vi "Convert Metadata Response to V1.vi"(8 "error in":errorcluster, 10 "get metadata response generic in":T10) -> (0 "error out":errorcluster, 2 "get metadata response v1 out":T1)   [LabVIEW 2020, in "Measurement Plugin Measurement Server.lvlib" / "Measurement Service V1.lvclass"]
uses:
  Measurement Service V1.lvclass
  Helpers/TypeDefs/Get Metadata Response.ctl
  Helpers/TypeDefs/Measurement Details.ctl
  Helpers/TypeDefs/Measurement Signature.ctl
  Helpers/TypeDefs/Configuration Parameter.ctl
  Helpers/TypeDefs/Parameter Annotations Entry.ctl
  <vilib>/gRPC/LabVIEW gRPC Library/Shared/Any.ctl
  Helpers/TypeDefs/Output Parameter.ctl
  Helpers/TypeDefs/User Interface Details.ctl
  Generated/Measurement Plugin Measurement Server Internal/RPC Messages/ni_measurementlink_measurement_v1_GetMetadataResponse.ctl
  Generated/Measurement Plugin Measurement Server Internal/RPC Messages/ni_measurementlink_measurement_v1_MeasurementDetails.ctl
  Generated/Measurement Plugin Measurement Server Internal/RPC Messages/ni_measurementlink_measurement_v1_MeasurementSignature.ctl
  Generated/Measurement Plugin Measurement Server Internal/RPC Messages/ni_measurementlink_measurement_v1_ConfigurationParameter.ctl
  Generated/Measurement Plugin Measurement Server Internal/RPC Messages/google_protobuf_Field_Kind.ctl
  Generated/Measurement Plugin Measurement Server Internal/RPC Messages/ni_measurementlink_measurement_v1_ConfigurationParameter_AnnotationsEntry.ctl
  Generated/Measurement Plugin Measurement Server Internal/RPC Messages/google_protobuf_Any.ctl
  Generated/Measurement Plugin Measurement Server Internal/RPC Messages/ni_measurementlink_measurement_v1_Output.ctl
  Generated/Measurement Plugin Measurement Server Internal/RPC Messages/ni_measurementlink_measurement_v1_UserInterfaceDetails.ctl
  Generated/Measurement Plugin Measurement Server Internal/Measurement Plugin Measurement Server Internal.lvlib
  Measurement Plugin Measurement Server.lvlib
  <vilib>/gRPC/LabVIEW gRPC Library/grpc-lvsupport-release.lvlib
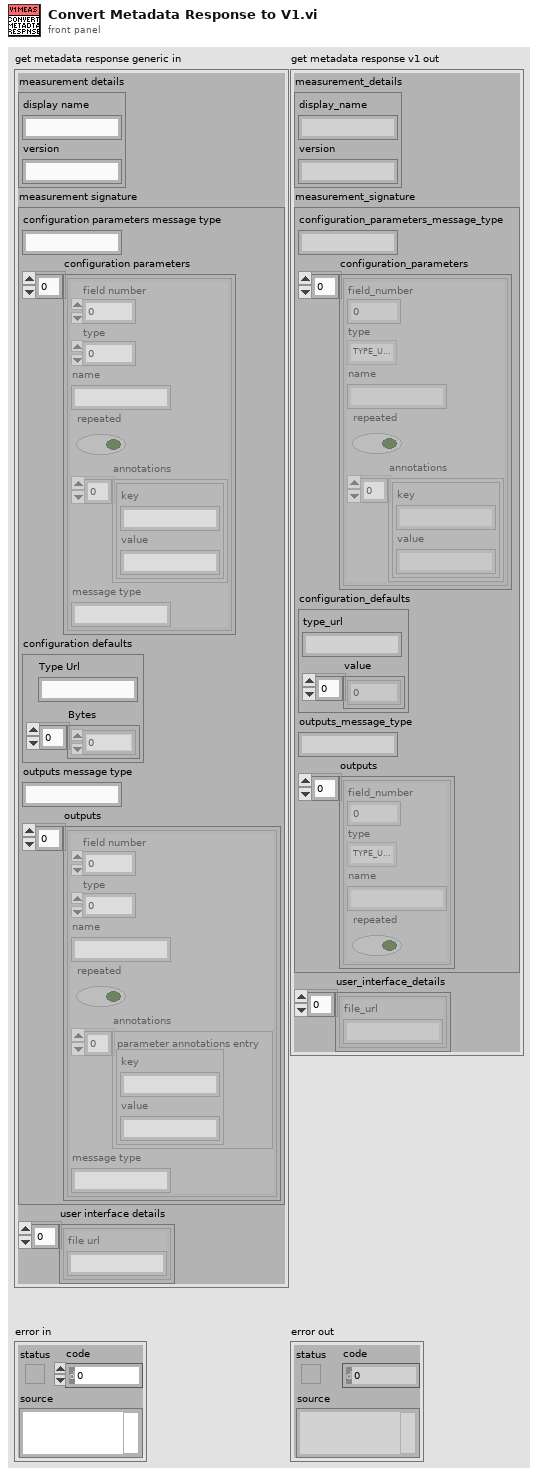
[diagram p1: front panel]
types:
  T1 = typedef "Measurement Plugin Measurement Server Internal.lvlib/ni_measurementlink_measurement_v1_GetMetadataResponse.ctl" = cluster{"measurement_details":T2, "measurement_signature":T3, "user_interface_details":T9[]}
  T2 = typedef "Measurement Plugin Measurement Server Internal.lvlib/ni_measurementlink_measurement_v1_MeasurementDetails.ctl" = cluster{"display_name":string, "version":string}
  T3 = typedef "Measurement Plugin Measurement Server Internal.lvlib/ni_measurementlink_measurement_v1_MeasurementSignature.ctl" = cluster{"configuration_parameters_message_type":string, "configuration_parameters":T4[], "configuration_defaults":T7, "outputs_message_type":string, "outputs":T8[]}
  T4 = typedef "Measurement Plugin Measurement Server Internal.lvlib/ni_measurementlink_measurement_v1_ConfigurationParameter.ctl" = cluster{"field_number":i32, "type":T5, "name":string, "repeated":bool, "annotations":T6[]}
  T5 = typedef "Measurement Plugin Measurement Server Internal.lvlib/google_protobuf_Field_Kind.ctl" = enum32{"TYPE_UNKNOWN", "TYPE_DOUBLE", "TYPE_FLOAT", "TYPE_INT64", "TYPE_UINT64", "TYPE_INT32", "TYPE_FIXED64", "TYPE_FIXED32", "TYPE_BOOL", "TYPE_STRING", "TYPE_GROUP", "TYPE_MESSAGE", "TYPE_BYTES", "TYPE_UINT32", "TYPE_ENUM", "TYPE_SFIXED32", "TYPE_SFIXED64", "TYPE_SINT32", "TYPE_SINT64"}
  T6 = typedef "Measurement Plugin Measurement Server Internal.lvlib/ni_measurementlink_measurement_v1_ConfigurationParameter_AnnotationsEntry.ctl" = cluster{"key":string, "value":string}
  T7 = typedef "Measurement Plugin Measurement Server Internal.lvlib/google_protobuf_Any.ctl" = cluster{"type_url":string, "value":u8[]}
  T8 = typedef "Measurement Plugin Measurement Server Internal.lvlib/ni_measurementlink_measurement_v1_Output.ctl" = cluster{"field_number":i32, "type":T5, "name":string, "repeated":bool}
  T9 = typedef "Measurement Plugin Measurement Server Internal.lvlib/ni_measurementlink_measurement_v1_UserInterfaceDetails.ctl" = cluster{"file_url":string}
  T10 = typedef "Measurement Plugin Measurement Server.lvlib/Get Metadata Response.ctl" = cluster{"measurement details":T11, "measurement signature":T12, "user interface details":T17[]}
  T11 = typedef "Measurement Plugin Measurement Server.lvlib/Measurement Details.ctl" = cluster{"display name":string, "version":string}
  T12 = typedef "Measurement Plugin Measurement Server.lvlib/Measurement Signature.ctl" = cluster{"configuration parameters message type":string, "configuration parameters":T13[], "configuration defaults":T15, "outputs message type":string, "outputs":T16[]}
  T13 = typedef "Measurement Plugin Measurement Server.lvlib/Configuration Parameter.ctl" = cluster{"field number":i32, "type":i32, "name":string, "repeated":bool, "annotations":T14[], "message type":string}
  T14 = typedef "Measurement Plugin Measurement Server.lvlib/Parameter Annotations Entry.ctl" = cluster{"key":string, "value":string}
  T15 = typedef "grpc-lvsupport-release.lvlib/Any.ctl" = cluster{"Type Url":string, "Bytes":u8[]}
  T16 = typedef "Measurement Plugin Measurement Server.lvlib/Output Parameter.ctl" = cluster{"field number":i32, "type":i32, "name":string, "repeated":bool, "annotations":T14[], "message type":string}
  T17 = typedef "Measurement Plugin Measurement Server.lvlib/User Interface Details.ctl" = cluster{"file url":string}
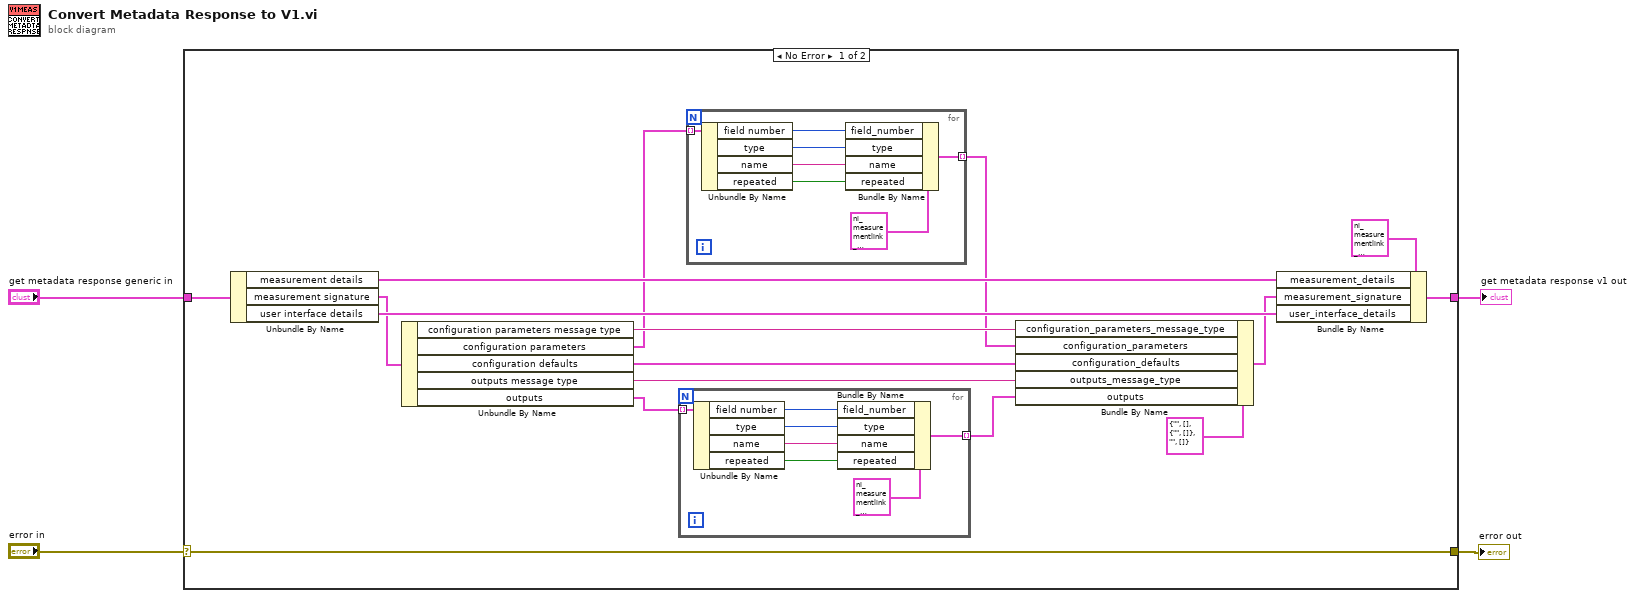
[diagram p0: block diagram]
diagram:
  n1 = case shown="No Error" "error in" {
    selector: "error in" -> [w20 w35]
    tunnel: [w20 w35] -> w3
    tunnel: "get metadata response generic in" -> [w19 _]
    tunnel: [w15 _] -> w1
    frame No Error {
      n2 = Unbundle By Name(w19) -> ("measurement details"=w17:T11, "measurement signature"=w13:T12, "user interface details"=w16:T17[])
      n3 = Unbundle By Name(w13) -> ("configuration parameters message type"=w12:string, "configuration parameters"=w6:T13[], "configuration defaults"=w11:T15, "outputs message type"=w10:string, "outputs"=w9:T16[])
      n4 = for {
        tunnel: w9 -> [w34] mode=indexing
        tunnel: [w28] -> w8 mode=indexing
        n5 = Unbundle By Name(w34) -> ("field number"=w32:i32, "type"=w31:i32, "name"=w30:string, "repeated"=w29:bool)
        n6 = Bundle By Name(cluster=T8 {"field_number"=0, "type"=enum."TYPE_UNKNOWN", "name"="", "repeated"=FALSE} ("ni_measurementlink_measurement_v1_Output"), "field_number"=w32, "type"=w31, "name"=w30, "repeated"=w29) -> (w28:T8)
      }
      n7 = for {
        tunnel: w6 -> [w27] mode=indexing
        tunnel: [w22] -> w5 mode=indexing
        n8 = Unbundle By Name(w27) -> ("field number"=w26:i32, "type"=w25:i32, "name"=w24:string, "repeated"=w23:bool)
        n9 = Bundle By Name(cluster=T4 {"field_number"=0, "type"=enum."TYPE_UNKNOWN", "name"="", "repeated"=FALSE, "annotations"=[]} ("ni_measurementlink_measurement_v1_ConfigurationParameter"), "field_number"=w26, "type"=w25, "name"=w24, "repeated"=w23) -> (w22:T4)
      }
      n10 = Bundle By Name(cluster=T3 {"configuration_parameters_message_type"="", "configuration_parameters"=[], "configuration_defaults"={"type_url"="", "value"=[]}, "outputs_message_type"="", "outputs"=[]} ("measurement_signature"), "configuration_parameters_message_type"=w12, "configuration_parameters"=w5, "configuration_defaults"=w11, "outputs_message_type"=w10, "outputs"=w8) -> (w7:T3)
      n11 = Bundle By Name(cluster=T1 {"measurement_details"={"display_name"="", "version"=""}, "measurement_signature"={"configuration_parameters_message_type"="", "configuration_parameters"=[], "configuration_defaults"={"type_url"="", "value"=[]}, "outputs_message_type"="", "outputs"=[]}, "user_interface_details"=[]} ("GetMetadataResponse V1 out"), "measurement_details"=w17, "measurement_signature"=w7, "user_interface_details"=w16) -> (w15:T1)
    }
    frame Error {
    }
  }
  "error out" <- w3
  "get metadata response v1 out" <- w1
